vi "HXG2_PGLY Q.vi"(0 "Liq In Avg. (°F)":dbl, 5 "Liq Out Avg. (°F)":dbl, 9 "Liq Flow (lbm/hr)":dbl, 11 "error in (no error)":errorcluster) -> (4 "Q Wtr (BTU/hr)":dbl, 6 "Cp (btu/lb)":dbl, 8 "Density (lbm/ft³)":dbl, 10 "Q Wtr (W)":dbl, 14 "mu (lbm/ft*s)":dbl, 15 "error out":errorcluster)   [LabVIEW 2012]
doc: "This VI calculates heat load for PGLY at the density specified. It uses another VI to calculate PGLY properties at the mean temperature."
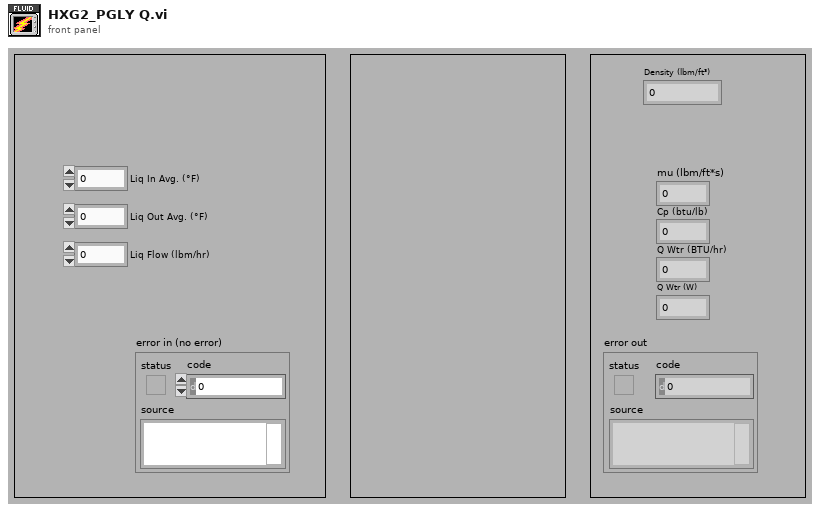
[diagram p1: front panel]
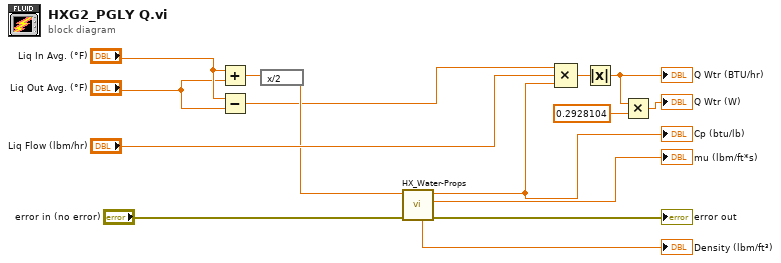
[diagram p0: block diagram]
diagram:
  n1 = Add(x="Liq In Avg. (°F)", y="Liq Out Avg. (°F)") -> (x+y=w3:dbl)
  n2 = Subtract(x="Liq In Avg. (°F)", y="Liq Out Avg. (°F)") -> (x-y=w1:dbl)
  n3 = expression code="x/2"(w3) -> (w2:dbl)
  n4 = call "HX_Water-Props.vi"("error in (no error)"="error in (no error)", "Water Avg (°F)"=w2) -> ("error out"=→"error out":errorcluster, "mu (lbm/ft*s)"=→"mu (lbm/ft*s)":dbl, "Cp (BTU/lbm°F)"=w10:dbl, "Density (lbm/ft³)"=→"Density (lbm/ft³)":dbl)  [unwired: 6 in]
  "Cp (btu/lb)" <- w10
  n5 = Compound Arithmetic op=MULTIPLY(w1, "Liq Flow (lbm/hr)", w10) -> (w5:dbl)
  n6 = Absolute Value(x=w5) -> (abs(x)=w7:dbl)
  "Q Wtr (BTU/hr)" <- w7
  n7 = Multiply(x=w7, y=0.2928104) -> (x*y=→"Q Wtr (W)":dbl)
